vi "Fin_GlobalVi.vi"() -> ()   [LabVIEW 2015]
panel:
  out "ChoosePanel":bool
  out "GlueSideUp":bool
  out "HV":bool
  in  "dimbar":T1={"top"=0, "left"=235, "bottom"=900, "right"=1024}
  in  "dimvertmenu":T1={"top"=0, "left"=0, "bottom"=900, "right"=235}
  in  "dimsmall":T1={"top"=0, "left"=235, "bottom"=650, "right"=1024}
  in  "dimbig":T1={"top"=0, "left"=235, "bottom"=900, "right"=1024}
  out "GlueSideDown":bool
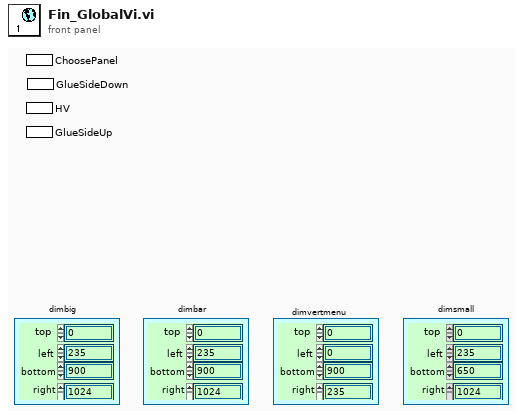
[diagram p1: front panel]
types:
  T1 = cluster{"top":i32, "left":i32, "bottom":i32, "right":i32}
diagram:
